vi "Check If Open VI Selected.vi"(9 "Drive Selection":T2, 10 "Open VI Folder Info":T1) -> (2 "Open VI Selected":bool, 3 "Open VI Path":path)   [LabVIEW 2014]
uses:
  Controls/Open VI Folder Info.ctl
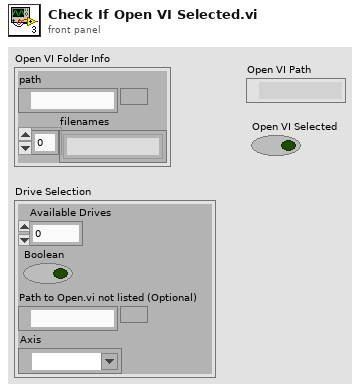
[diagram p1: front panel]
types:
  T1 = typedef "Open VI Folder Info.ctl" = cluster{"path":path, "filenames":string[]}
  T2 = cluster{"Available Drives":i32, "Boolean":bool, "Path to Open.vi not listed (Optional)":path, "Axis":refnum<k21>}
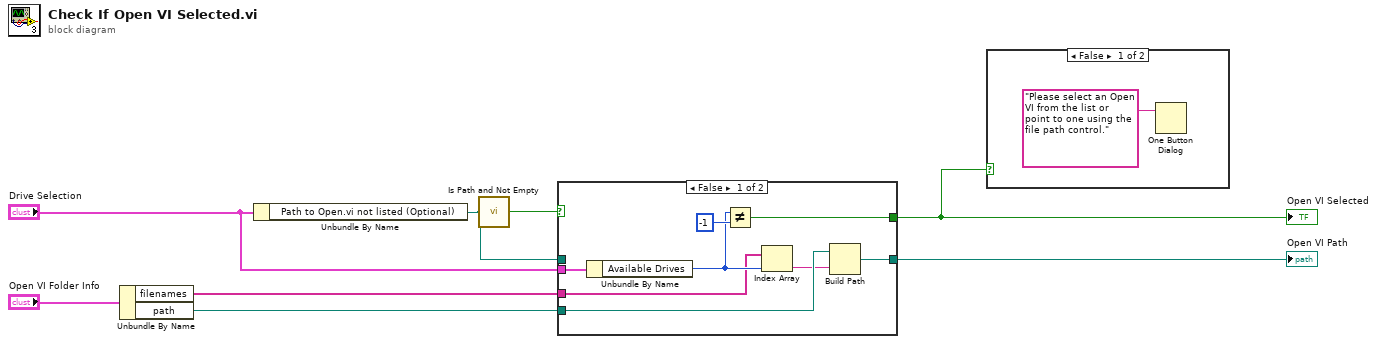
[diagram p0: block diagram]
diagram:
  n1 = Unbundle By Name("Open VI Folder Info") -> ("filenames"=w3:string[], "path"=w2:path)
  n2 = Unbundle By Name("Drive Selection") -> ("Path to Open.vi not listed (Optional)"=w5:path)
  n3 = call <vilib>:"Is Path and Not Empty.vi"("path"=w5) -> ("Is Path and Not Empty?"=w6:bool)  [unwired: 4 in]
  n4 = case shown="False" w6 {
    selector: w6 -> [_ w18]
    tunnel: [w16 w17] -> w8
    tunnel: [w15 w18] -> w1
    tunnel: "Drive Selection" -> [w12 _]
    tunnel: w3 -> [w11 _]
    tunnel: w2 -> [w10 _]
    tunnel: w5 -> [_ w17]
    frame False {
      n5 = Unbundle By Name(w12) -> ("Available Drives"=w13:i32)
      n6 = Not Equal?(x=w13, y=-1) -> (x != y?=w15:bool)
      n7 = Index Array(array=w11, index=w13) -> (element=w9:string)
      n8 = Build Path(base path=w10, name or relative path=w9) -> (appended path=w16:path)
    }
    frame True {
    }
  }
  "Open VI Path" <- w8
  "Open VI Selected" <- w1
  n9 = case shown="False" w1 {
    frame False {
      n10 = One Button Dialog(message="Please select an Open VI from the list or point to one using the file path control.") -> ()  [unwired: 1 in, 1 out]
    }
    frame True {
    }
  }
